vi "selectSummaryDataAll.vi"(8 "Shift":string="中", 10 "End_date":string="2014/11/13", 11 "Begin_date":string="2014/11/12") -> (2 "Summary":string[][](array[string]))   [LabVIEW 2012]
uses:
  <vilib>/addons/database/Auxilliary.llb/DB Tools Cursor Type.ctl
  <vilib>/addons/database/Connection.llb/DB Tools Open Connec (Path).vi
  <vilib>/addons/database/Connection.llb/Conn Execute.vi
  <vilib>/addons/database/Recordset.llb/Rec Fetch Recordset Data (R).vi
  <vilib>/addons/database/Recordset.llb/Rec Destroy - Connection.vi
  <vilib>/addons/database/_DB Variant To Data/Database Variant To Data.xnode
  <vilib>/addons/database/NI_Database_API.lvlib
panel:
  out "concatenated string":string
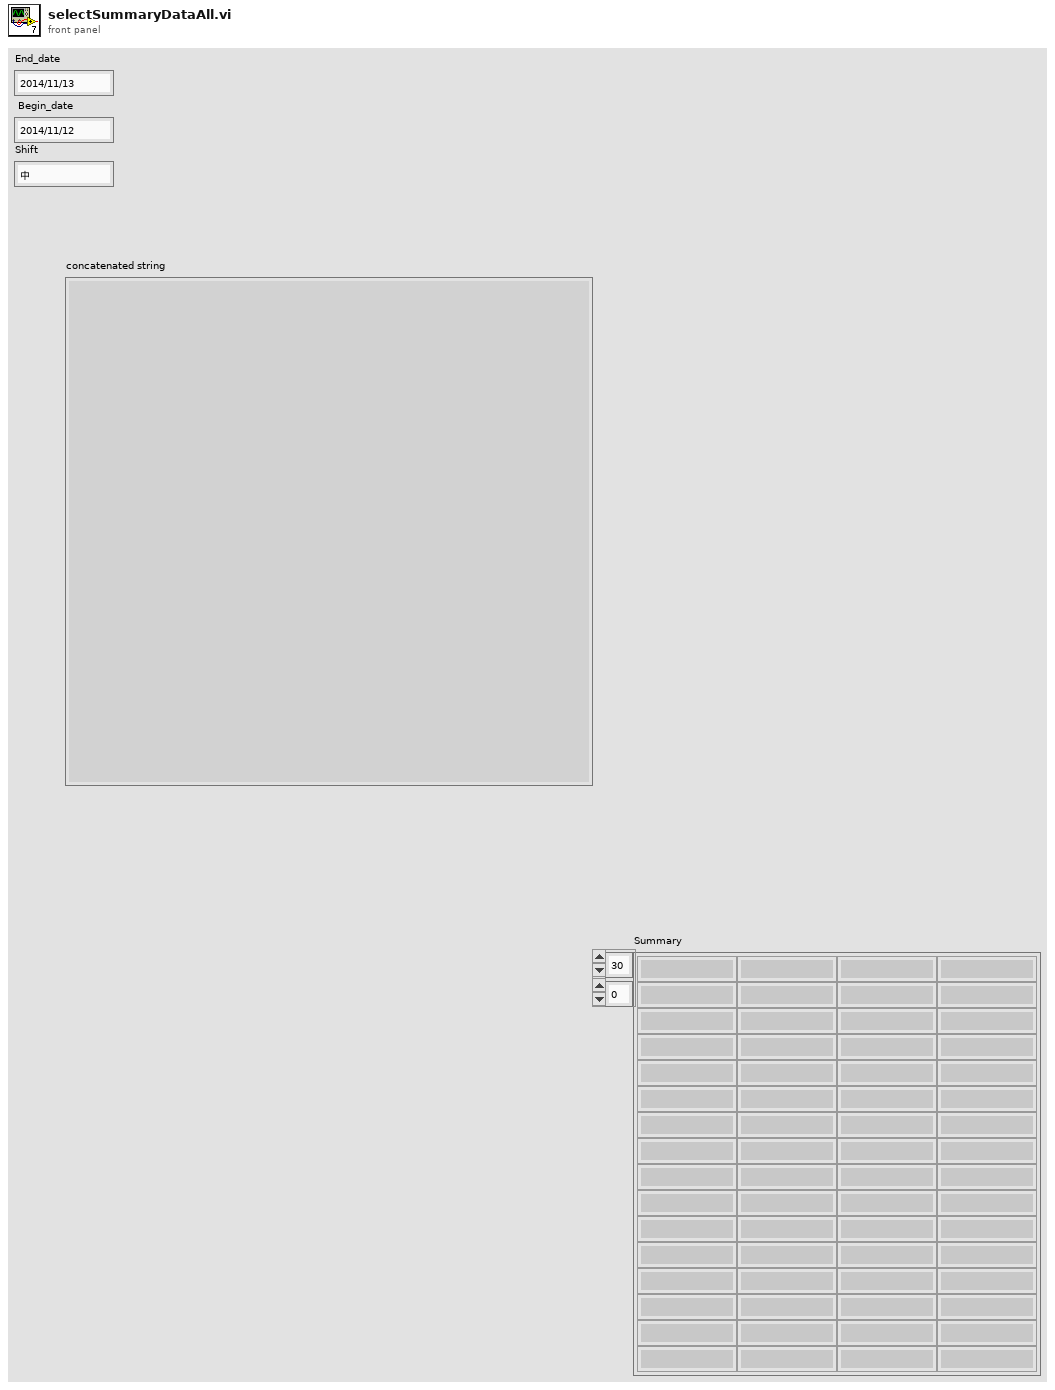
[diagram p1: front panel]
types:
  T1 = typedef "NI_Database_API.lvlib/DB Tools Cursor Type.ctl" = enum16{"forward-only", "keyset", "dynamic", "static"}
  T2 = typedef "NI_Database_API.lvlib/Conn ObjectReference.ctl" = refnum<k1>
  T3 = typedef "NI_Database_API.lvlib/Rec ObjectReference.ctl" = refnum<k1>
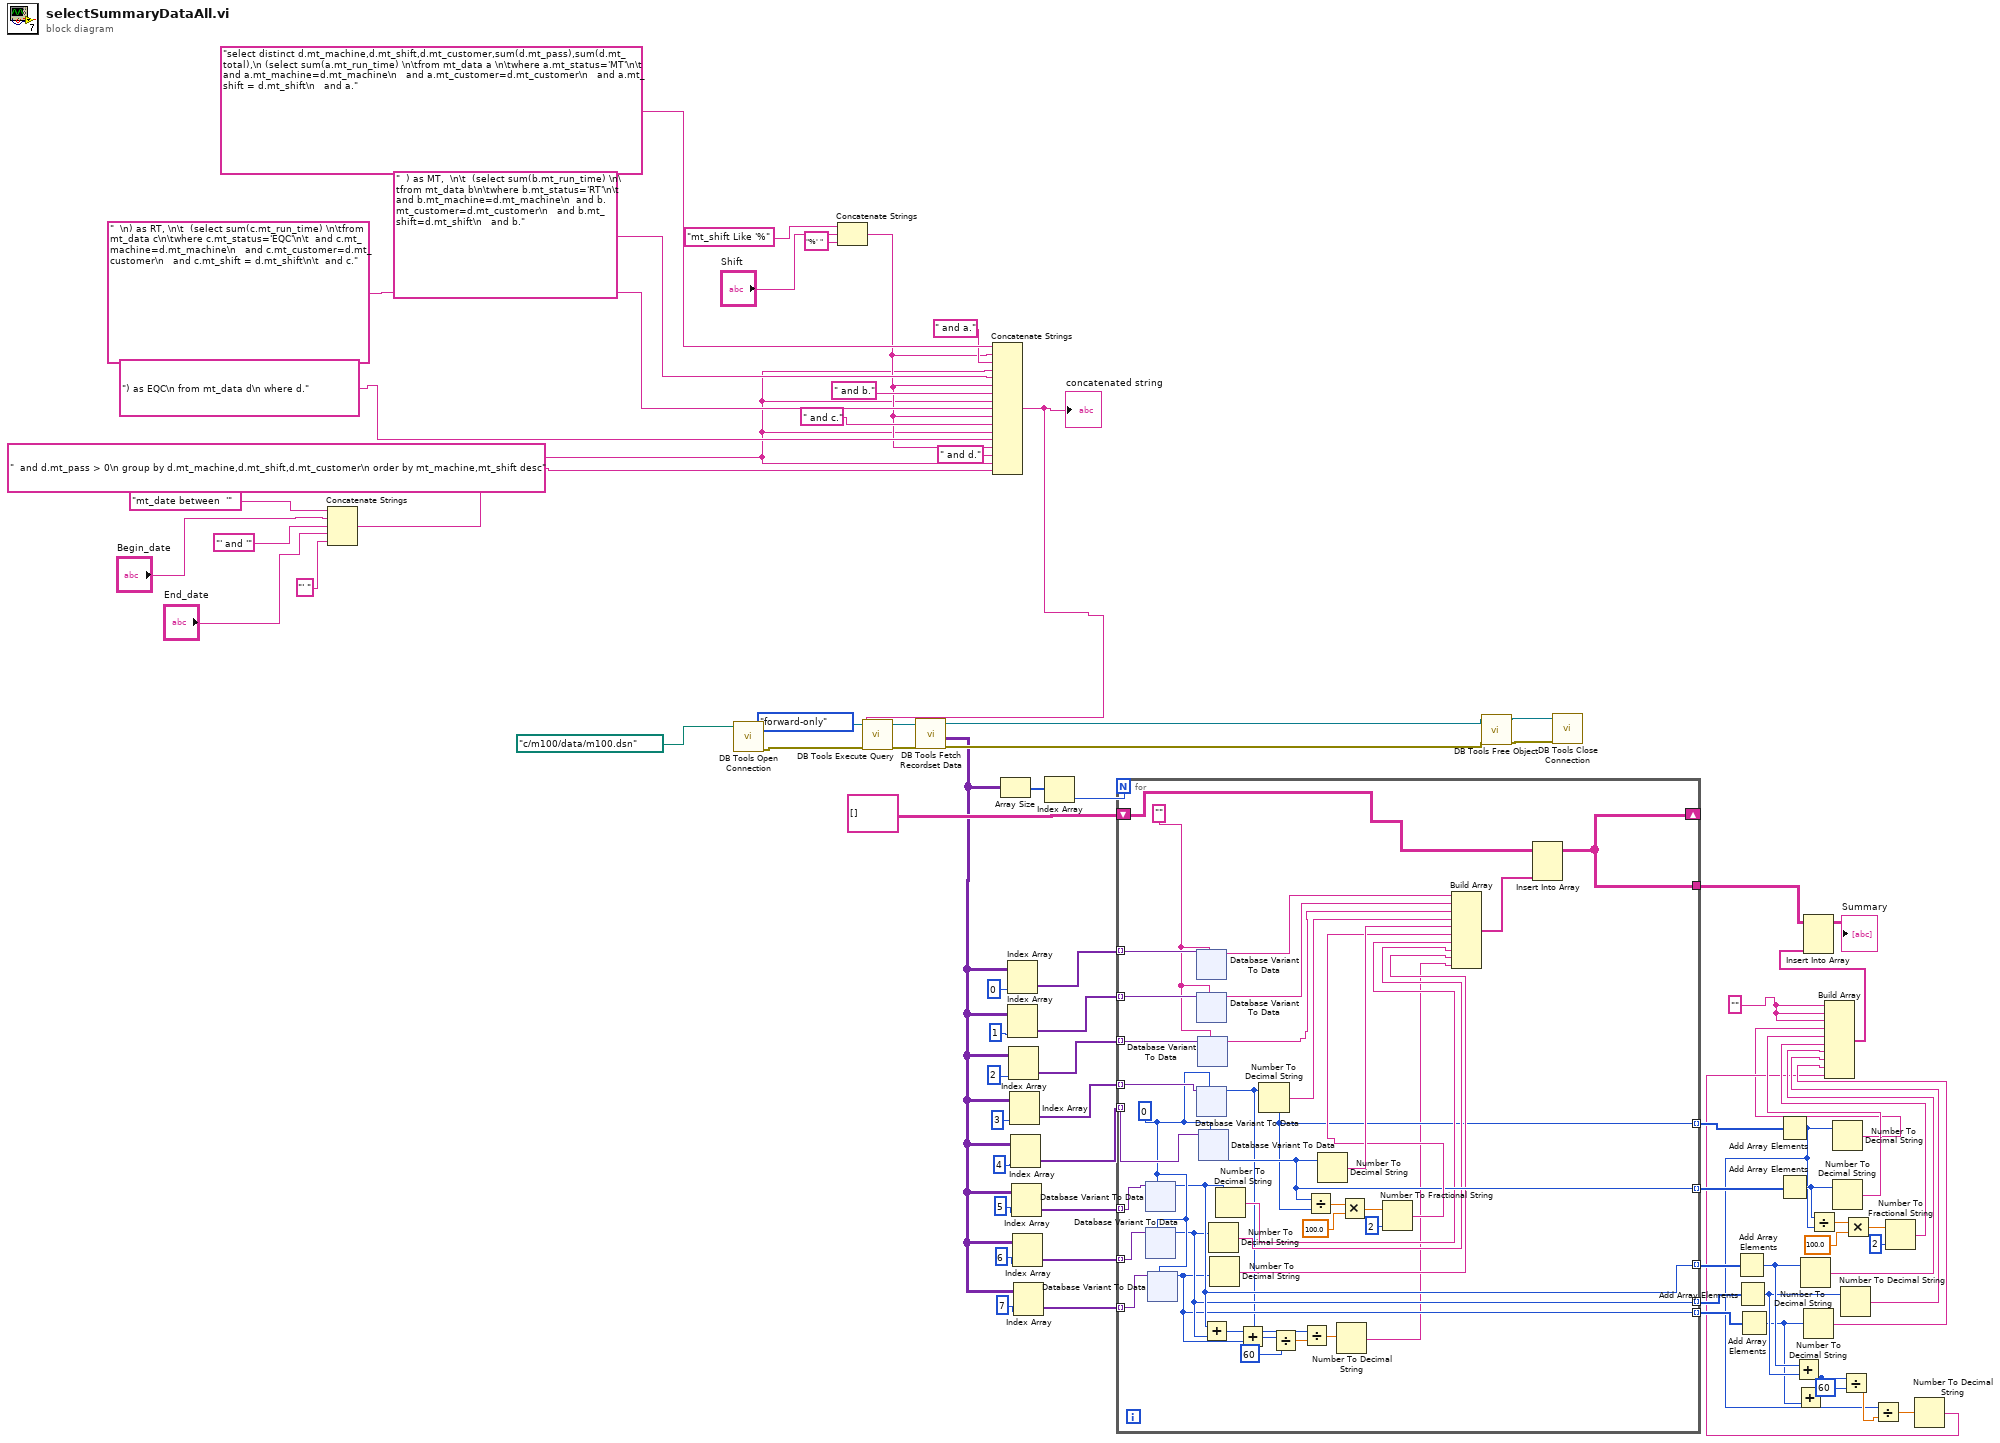
[diagram p0: block diagram]
diagram:
  w63 = "" ("element")
  n1 = Concatenate Strings("mt_date between  '", "Begin_date", "' and '" ("string"), "End_date", "' " ("string")) -> (w4:string)
  n2 = call-poly <vilib>:"DB Tools Open Connection.vi"("connection information"=path "c:/m100/data/m100.dsn") -> ("error out"=w51:errorcluster, "connection reference"=w52:T2)  [unwired: 7 in]
  n3 = Concatenate Strings("mt_shift Like '%" ("string"), "Shift", "%' " ("string")) -> (w6:string)
  n4 = Concatenate Strings("select distinct d.mt_machine,d.mt_shift,d.mt_customer,sum(d.mt_pass),sum(d.mt_total),\n (select sum(a.mt_run_time) \n\tfrom mt_data a \n\twhere a.mt_status='MT'\n\t  and a.mt_machine=d.mt_machine\n   and a.mt_customer=d.mt_customer\n   and a.mt_shift = d.mt_shift\n   and a." ("string"), w6, " and a." ("string"), w4, "  ) as MT,  \n\t  (select sum(b.mt_run_time) \n\tfrom mt_data b\n\twhere b.mt_status='RT'\n\t  and b.mt_machine=d.mt_machine\n  and b.mt_customer=d.mt_customer\n   and b.mt_shift=d.mt_shift\n   and b." ("string"), w6, " and b." ("string"), w4, "  \n) as RT, \n\t  (select sum(c.mt_run_time) \n\tfrom mt_data c\n\twhere c.mt_status='EQC'\n\t  and c.mt_machine=d.mt_machine\n   and c.mt_customer=d.mt_customer\n   and c.mt_shift = d.mt_shift\n\t  and c." ("string"), w6, " and c." ("string"), w4, ") as EQC\n from mt_data d\n where d." ("string"), w6, " and d." ("string"), w4, "  and d.mt_pass > 0\n group by d.mt_machine,d.mt_shift,d.mt_customer\n order by mt_machine,mt_shift desc" ("string")) -> (w1:string)
  "concatenated string" <- w1
  n5 = call-poly <vilib>:"DB Tools Execute Query.vi"("error in (no error)"=w51, "cursor type"=DB_Tools_Cursor_Type."forward-only", "SQL query"=w1, "connection reference"=w52) -> ("error out"=w54:errorcluster, "recordset reference"=w53:T3)  [unwired: 4 in]
  n6 = call-poly <vilib>:"DB Tools Fetch Recordset Data.vi"("error in (no error)"=w54, "recordset reference"=w53) -> ("error out"=w50:errorcluster, "recordset data"=w43:variant[][], "recordset reference out"=w49:T3)  [unwired: 3 in]
  n7 = Array Size(array=w43) -> (size(s)=w79:i32[])
  n8 = Index Array(array=w43, index (col)=0) -> (element=w72:variant[])  [unwired: 1 in]
  n9 = Index Array(array=w43, index (col)=1) -> (element=w71:variant[])  [unwired: 1 in]
  n10 = Index Array(array=w43, index (col)=2) -> (element=w67:variant[])  [unwired: 1 in]
  n11 = Index Array(array=w43, index (col)=3) -> (element=w70:variant[])  [unwired: 1 in]
  n12 = Index Array(array=w43, index (col)=4) -> (element=w69:variant[])  [unwired: 1 in]
  n13 = Index Array(array=w43, index (col)=5) -> (element=w42:variant[])  [unwired: 1 in]
  n14 = Index Array(array=w43, index (col)=6) -> (element=w41:variant[])  [unwired: 1 in]
  n15 = Index Array(array=w43, index (col)=7) -> (element=w40:variant[])  [unwired: 1 in]
  n16 = Index Array(array=w79) -> (element=w78:i32)  [unwired: 1 in]
  n17 = for {
    N: w78 -> [_]
    tunnel: w69 -> [w116] mode=indexing
    shift-right: [w97] -> _
    shift-left: string[][] [] -> [w101]
    tunnel: w72 -> [w115] mode=indexing
    tunnel: w71 -> [w114] mode=indexing
    tunnel: w70 -> [w113] mode=indexing
    tunnel: w67 -> [w110] mode=indexing
    tunnel: [w82] -> w30 mode=indexing
    tunnel: [w103] -> w66 mode=indexing
    tunnel: [w97] -> w47
    tunnel: w42 -> [w96] mode=indexing
    tunnel: w41 -> [w95] mode=indexing
    tunnel: w40 -> [w94] mode=indexing
    tunnel: [w86] -> w37 mode=indexing
    tunnel: [w88] -> w38 mode=indexing
    tunnel: [w89] -> w39 mode=indexing
    w93 = 0
    w109 = ""
    n18 = xnode "Database Variant To Data"("database variant"=w96, "type"=w93) -> ("data"=w89:i32)  [unwired: 1 in, 1 out]
    n19 = xnode "Database Variant To Data"("database variant"=w95, "type"=w93) -> ("data"=w88:i32)  [unwired: 1 in, 1 out]
    n20 = xnode "Database Variant To Data"("database variant"=w94, "type"=w93) -> ("data"=w86:i32)  [unwired: 1 in, 1 out]
    n21 = xnode "Database Variant To Data"("database variant"=w115, "type"=w109) -> ("data"=w100:string)  [unwired: 1 in, 1 out]
    n22 = xnode "Database Variant To Data"("database variant"=w114, "type"=w109) -> ("data"=w99:string)  [unwired: 1 in, 1 out]
    n23 = xnode "Database Variant To Data"("database variant"=w113, "type"=w93) -> ("data"=w82:i32)  [unwired: 1 in, 1 out]
    n24 = xnode "Database Variant To Data"("database variant"=w110, "type"=w109) -> ("data"=w98:string)  [unwired: 1 in, 1 out]
    n25 = xnode "Database Variant To Data"("database variant"=w116, "type"=w93) -> ("data"=w103:i32)  [unwired: 1 in, 1 out]
    n26 = Add(x=w89, y=w88) -> (x+y=w87:i32)
    n27 = Number To Decimal String(number=w88) -> (decimal integer string=w91:string)  [unwired: 1 in]
    n28 = Number To Decimal String(number=w86) -> (decimal integer string=w90:string)  [unwired: 1 in]
    n29 = Number To Decimal String(number=w89) -> (decimal integer string=w92:string)  [unwired: 1 in]
    n30 = Add(x=w87, y=w86) -> (x+y=w85:i32)
    n31 = Number To Decimal String(number=w82) -> (decimal integer string=w107:string)  [unwired: 1 in]
    n32 = Divide(x=w85, y=60) -> (x/y=w83:dbl)
    n33 = Divide(x=w82, y=w83) -> (x/y=w81:dbl)
    n34 = Divide(x=w103, y=w82) -> (x/y=w111:dbl)
    n35 = Number To Decimal String(number=w103) -> (decimal integer string=w108:string)  [unwired: 1 in]
    n36 = Number To Decimal String(number=w81) -> (decimal integer string=w80:string)  [unwired: 1 in]
    n37 = Multiply(x=w111, y=100.0) -> (x*y=w106:dbl)
    n38 = Number To Fractional String(number=w106, precision (6)=i16 2) -> (F-format string=w105:string)  [unwired: 2 in]
    n39 = Build Array(w100, w99, w98, w107, w108, w105, w92, w91, w90, w80) -> (w102:string[])
    n40 = Insert Into Array(array=w101, new element=w102) -> (w97:string[][])  [unwired: 2 in]
  }
  n41 = call-poly <vilib>:"DB Tools Free Object.vi"("error in (no error)"=w50, "recordset reference"=w49) -> ("error out"=w55:errorcluster, "connection reference"=w56:T2)  [unwired: 8 in]
  n42 = call <vilib>:"DB Tools Close Connection.vi"("error in (no error)"=w55, "connection reference"=w56) -> ()  [unwired: 5 in, 1 out]
  n43 = Add Array Elements(numeric array=w39) -> (sum=w33:i32)
  n44 = Add Array Elements(numeric array=w38) -> (sum=w32:i32)
  n45 = Add Array Elements(numeric array=w37) -> (sum=w31:i32)
  n46 = Add Array Elements(numeric array=w30) -> (sum=w24:i32)
  n47 = Add Array Elements(numeric array=w66) -> (sum=w58:i32)
  n48 = Add(x=w33, y=w32) -> (x+y=w29:i32)
  n49 = Add(x=w29, y=w31) -> ()  [unwired: 1 out]
  n50 = Number To Decimal String(number=w33) -> (decimal integer string=w36:string)  [unwired: 1 in]
  n51 = Number To Decimal String(number=w31) -> (decimal integer string=w34:string)  [unwired: 1 in]
  n52 = Divide(x=w58, y=w24) -> (x/y=w61:dbl)
  n53 = Number To Decimal String(number=w24) -> (decimal integer string=w23:string)  [unwired: 1 in]
  n54 = Number To Decimal String(number=w58) -> (decimal integer string=w65:string)  [unwired: 1 in]
  n55 = Number To Decimal String(number=w32) -> (decimal integer string=w35:string)  [unwired: 1 in]
  n56 = Divide(x=w29, y=60) -> (x/y=w27:dbl)
  n57 = Multiply(x=w61, y=100.0) -> (x*y=w60:dbl)
  n58 = Divide(x=w24, y=w27) -> (x/y=w26:dbl)
  n59 = Number To Fractional String(number=w60, precision (6)=i16 2) -> (F-format string=w57:string)  [unwired: 2 in]
  n60 = Number To Decimal String(number=w26) -> (decimal integer string=w25:string)  [unwired: 1 in]
  n61 = Build Array(w63, w63, w63, w23, w65, w57, w36, w35, w34, w25) -> (w64:string[])
  n62 = Insert Into Array(array=w47, new element=w64) -> (→"Summary":string[][])  [unwired: 2 in]
